vi "Read Parent Attributes.vi"(11 "Base Actor in":refnum<class "Base Actor.lvclass">) -> (2 "Parent Attributes":refnum<class "Attributes.lvclass">)   [LabVIEW 2025, in "jettl.lvlib" / "Actor.lvlib" / "Base Actor.lvclass"]
uses:
  Base Actor.lvclass
  Base Actor.lvclass/Base Actor.ctl
  Attributes/Attributes/Attributes.lvclass
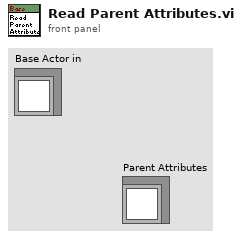
[diagram p1: front panel]
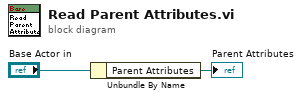
[diagram p0: block diagram]
diagram:
  n1 = Unbundle By Name("Base Actor in") -> ("Parent Attributes"=→"Parent Attributes":refnum<class "Attributes.lvclass">)
